vi "DemoHW_VI.vi"() -> (0 "STDEV":i32, 3 "Velocity (m/s)":dbl)   [LabVIEW 2017]
uses:
  <vilib>/Analysis/baseanly.llb/Mean (DBL).vi
  <vilib>/Analysis/NI_AALBase.lvlib
panel:
  out "Input Voltage":dbl
  out "Flow Meter (m/s)":i32(knob) scale=-50.0..50.0
  in  "Transducer Offset (V)":dbl
  # "Flow VI"
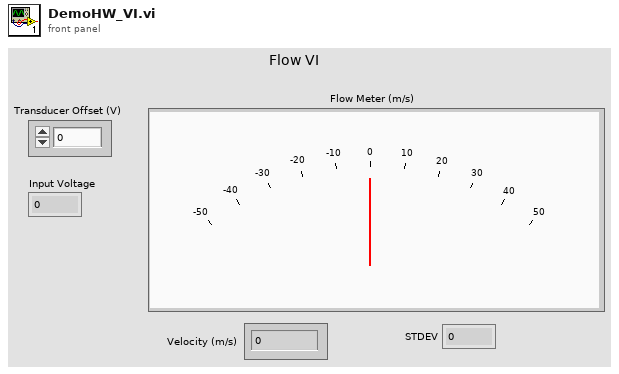
[diagram p1: front panel]
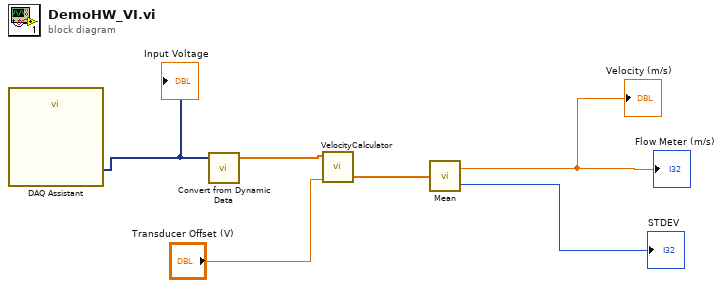
[diagram p0: block diagram]
diagram:
  n1 = call "DAQ Assistant"() -> ("data"=w3:dynamicdata)  [unwired: 17 in, 2 out]
  "Input Voltage" <- w3
  n2 = call "Convert from Dynamic Data"("Dynamic Data Type"=w3) -> ("Array"=w2:dbl[])  [unwired: 3 in]
  n3 = call "VelocityCalculator.vi"("Offset (V)"="Transducer Offset (V)", "Voltage Input"=w2) -> ("Veloctiy Output [m/s]"=w6:dbl[])  [unwired: 9 in]
  n4 = call-poly <vilib>:"Mean.vi"("X"=w6) -> ("mean"=→"Flow Meter (m/s)" →"Velocity (m/s)":dbl, "error"=→"STDEV":i32)
